vi "NIDCPower_channel_ganging - reset device.vi"(8 "error in (no error)":errorcluster, 11 "Ganged Session In":T1) -> (0 "error out":errorcluster, 3 "Ganged Session Out":T1)   [LabVIEW 2021]
uses:
  ctl/NIDCPower_channel_ganging - ctl - ganged config.ctl
  ctl/NIDCPower_channel_ganging - ctl - channel mode.ctl
  ctl/NIDCPower_channel_ganging - ctl - ganged session.ctl
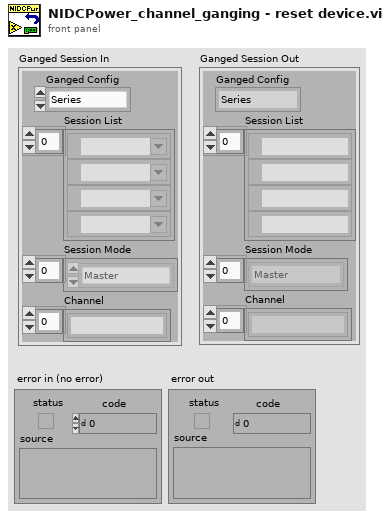
[diagram p1: front panel]
types:
  T1 = typedef "NIDCPower_channel_ganging - ctl - ganged session.ctl" = cluster{"Ganged Config":T2, "Session List":refnum<k15>[], "Session Mode":T3[], "Channel":string[]}
  T2 = typedef "NIDCPower_channel_ganging - ctl - ganged config.ctl" = enum16{"Series", "Parallel", "Manual"}
  T3 = typedef "NIDCPower_channel_ganging - ctl - channel mode.ctl" = enum16{"Master", "Slave", "Slave - Inverted"}
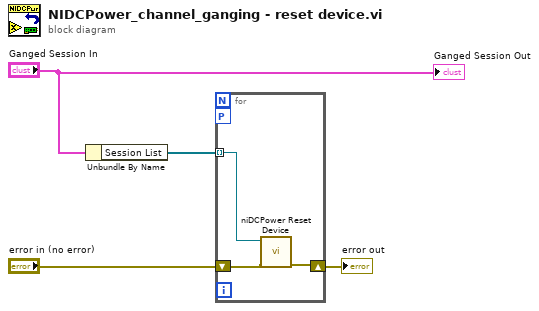
[diagram p0: block diagram]
diagram:
  n1 = Unbundle By Name("Ganged Session In") -> ("Session List"=w1:refnum<k15>[])
  n2 = for {
    shift-right: [w7] -> w3
    shift-left: "error in (no error)" -> [w6]
    tunnel: w1 -> [w5] mode=indexing
    workers-P: _ -> [_]
    n3 = call <instrlib>:"niDCPower Reset Device.vi"("error in (no error)"=w6, "instrument handle"=w5) -> ("error out"=w7:errorcluster)  [unwired: 8 in, 1 out]
  }
  "error out" <- w3
  "Ganged Session Out" <- "Ganged Session In"
